vi "StateArm.vi"(0 "Master State In":T1(ring)) -> ()   [LabVIEW 2020]
doc: "This VI makes all of the decisions related to the Arm subsystem."
uses:
  <vilib>/Rock Robotics/WPI/DriverStation/WPI_DriverStationRobotMode2.ctl
  91f446a8-b483-4e57-bb67-dcd3392c5748.vi
  cc244f82-53a2-44a0-9b94-e9a7b6ef83dd.vi
  GlobalDriverStationCommands.vi
  GlobalPoseAndTargeting.vi
  GlobalDriverStationData.vi
  GlobalArm.vi
panel:
  out "Pre-Ground":cluster{dbl, dbl, dbl}
  in  "Pre-Ground Auto":cluster{dbl, dbl, dbl}={113.0, 144.0, 280.0}
  in  "Pre-Scoring Mid Cube":cluster{dbl, dbl, dbl}={90.0, 180.0, 180.0}
  in  "Pre-Scoring High Cube":cluster{dbl, dbl, dbl}={100.0, 270.0, 109.0}
  in  "Pre-Scoring Mid Cone":cluster{dbl, dbl, dbl}={90.0, 280.0, 90.0}
  in  "Pre-Scoring High Cone":cluster{dbl, dbl, dbl}={100.0, 275.0, 85.0}
  in  "Ground":cluster{dbl, dbl, dbl}={113.0, 144.0, 350.0}
  in  "Pre-Substation":cluster{dbl, dbl, dbl}={80.0, 149.0, 215.0}
  in  "Low Score Back":cluster{dbl, dbl, dbl}={90.0, 180.0, 155.0}
  in  "Low Score Front":cluster{dbl, dbl, dbl}={90.0, 180.0, 265.0}
  in  "Shelf":cluster{dbl, dbl, dbl}={104.0, 290.0, -72.0}
  in  "High Cube (IK)":cluster{dbl, dbl, dbl}={202.0, -50.7, 59.0}
  in  "Mid Cube (IK)":cluster{dbl, dbl, dbl}={210.0, -35.5, 50.0}
  in  "High Cone (IK)":cluster{dbl, dbl, dbl}={190.0, -53.0, 62.5}
  in  "Mid Cone (IK)":cluster{dbl, dbl, dbl}={180.0, -42.5, 51.7}
  in  "Pre-Shelf":cluster{dbl, dbl, dbl}={104.0, 309.0, -85.0}
  in  "Initial Scoring Guess":cluster{dbl, dbl, dbl}={100.0, 230.0, 125.0}
  out "Current Sequence Step":i32
  in  "Substation":cluster{dbl, dbl, dbl}={80.0, 149.0, 280.0}
  in  "Stowed":cluster{dbl, dbl, dbl}={90.0, 180.0, 180.0}
  in  "Pre-Ground Teleop":cluster{dbl, dbl, dbl}={113.0, 144.0, 180.0}
  out "You Have Arrived":bool
  out "Pre-Scoring":cluster{dbl, dbl, dbl}
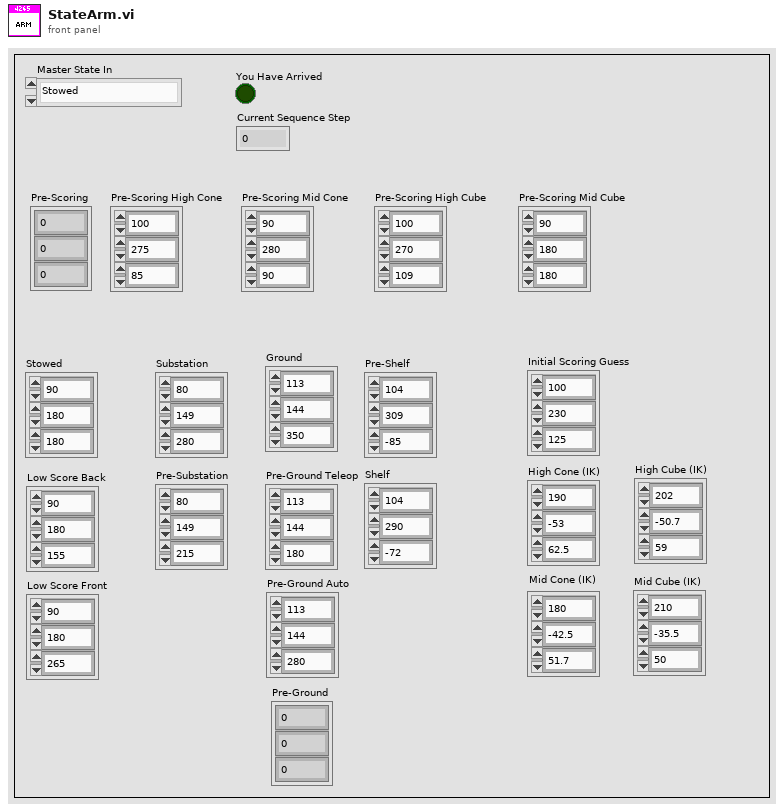
[diagram p1: front panel]
types:
  T1 = enum16{"Stowed", "Balancing", "Scoring", "Hoppering", "Ground", "Shelf"}
  T2 = typedef "WPI_DriverStationRobotMode2.ctl" = enum16{"Autonomous Disabled", "Autonomous Enabled", "Teleop Disabled", "Teleop Enabled", "Disconnected", "Finish", "Test Disabled", "Test Enabled", "Emergency Stopped"}
  T3 = enum16{"Low Cube", "Mid Cube", "High Cube", "Low Cone", "Mid Cone", "High Cone"}
  T4 = enum16{"Safety", "Travelling", "Positioning", "Holding"}
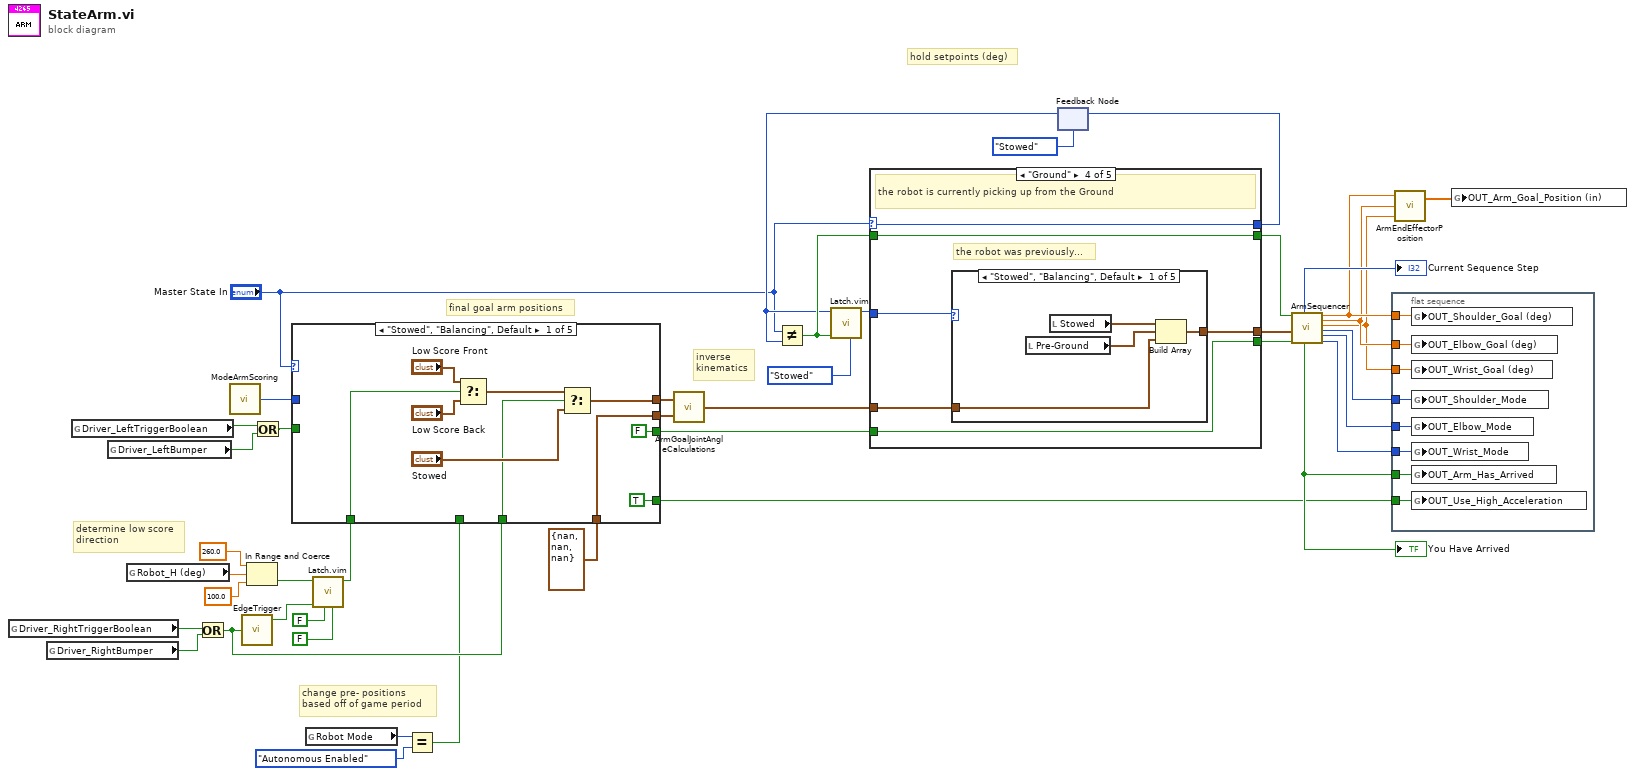
[diagram p0: block diagram]
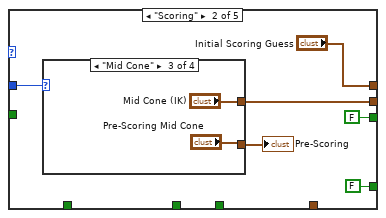
[diagram p2: hidden frame]
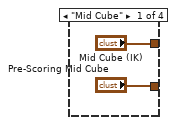
[diagram p3: hidden frame]
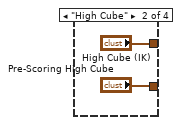
[diagram p4: hidden frame]
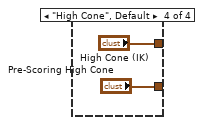
[diagram p5: hidden frame]
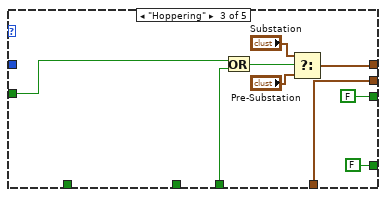
[diagram p6: hidden frame]
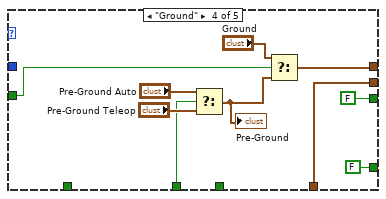
[diagram p7: hidden frame]
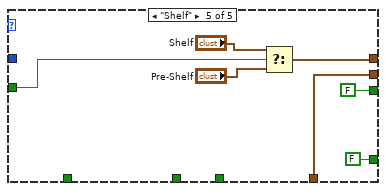
[diagram p8: hidden frame]
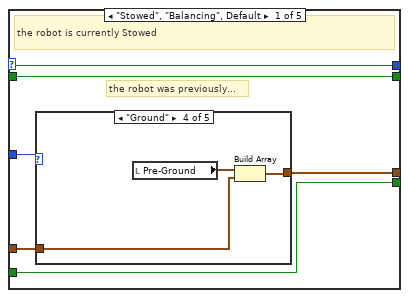
[diagram p9: hidden frame]
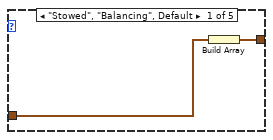
[diagram p10: hidden frame]
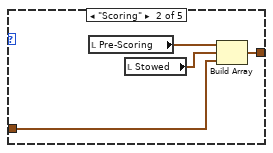
[diagram p11: hidden frame]
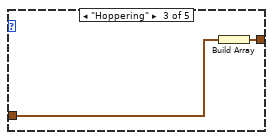
[diagram p12: hidden frame]
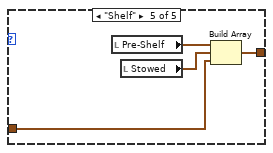
[diagram p13: hidden frame]
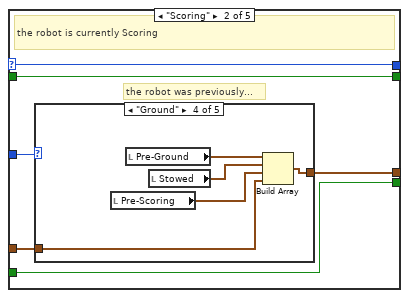
[diagram p14: hidden frame]
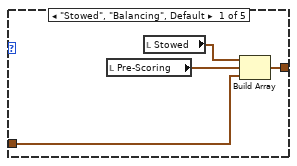
[diagram p15: hidden frame]
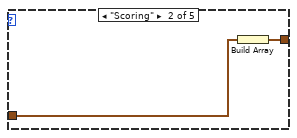
[diagram p16: hidden frame]
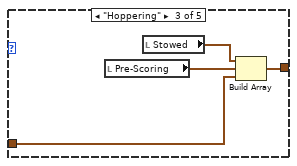
[diagram p17: hidden frame]
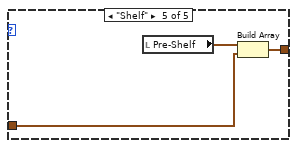
[diagram p18: hidden frame]
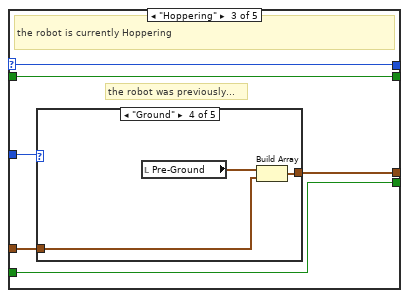
[diagram p19: hidden frame]
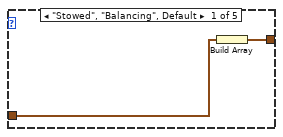
[diagram p20: hidden frame]
diagram:
  # "change pre- positions\nbased off of game period"
  # "determine low score\ndirection"
  # "inverse\nkinematics"
  # "hold setpoints (deg)"
  # "final goal arm positions"
  n1 = global read "GlobalDriverStationCommands.vi" "Driver_RightTriggerBoolean"() -> (w6:bool)
  n2 = global read "GlobalDriverStationCommands.vi" "Driver_RightBumper"() -> (w7:bool)
  n3 = global read "GlobalDriverStationCommands.vi" "Driver_LeftTriggerBoolean"() -> (w10:bool)
  n4 = global read "GlobalDriverStationCommands.vi" "Driver_LeftBumper"() -> (w9:bool)
  n5 = global read "GlobalPoseAndTargeting.vi" "Robot_H (deg)"() -> (w18:dbl)
  n6 = Or(x=w6, y=w7) -> (x .or. y?=w5:bool)
  n7 = call "ModeArmScoring.vi"() -> ("Scoring Position"=w28:T3)  [unwired: 1 in]
  n8 = call "EdgeTrigger.vi"("Input Signal"=w5) -> ("Rising Edge Trigger"=w12:bool)  [unwired: 2 out]
  n9 = In Range and Coerce(upper limit=260.0, x=w18, lower limit=100.0) -> (In Range?=w15:bool)  [unwired: 1 out]
  n10 = Or(x=w10, y=w9) -> (x .or. y?=w8:bool)
  n11 = global read "GlobalDriverStationData.vi" "Robot Mode"() -> (w4:T2)
  n12 = call "Latch.vim"("Default Value"=FALSE, "Reset"=FALSE, "Latch Signal"=w12, "Latch Value"=w15) -> ("Latched"=w11:bool)  [unwired: 7 in]
  n13 = Equal?(x=w4, y=WPI_DriverStationRobotMode2."Autonomous Enabled") -> (x = y?=w2:bool)
  n14 = case shown="\"Stowed\", \"Balancing\", Default" "Master State In" {
    tunnel: w28 -> [_ w59 _ _ _]
    tunnel: [w47 "Initial Scoring Guess" w73 w84 w89] -> w30
    tunnel: [w53 w58 w76 w86 w90] -> w27
    tunnel: cluster{dbl, dbl, dbl} {nan, nan, nan} ("PreShelf (IK)") -> [w53 _ w76 w86 w90]
    tunnel: [FALSE ("OUT_Hopper_Arm_Position") FALSE ("OUT_Hopper_Arm_Position") FALSE ("OUT_Hopper_Arm_Position") FALSE ("OUT_Hopper_Arm_Position") FALSE ("OUT_Hopper_Arm_Position")] -> w20
    tunnel: w11 -> [w46 _ _ _ _]
    tunnel: w5 -> [w45 _ w70 _ _]
    tunnel: w8 -> [_ _ w69 w82 w88]
    tunnel: w2 -> [_ _ _ w78 _]
    tunnel: [TRUE FALSE FALSE FALSE FALSE] -> w1
    frame "Stowed", "Balancing", Default {
      n15 = Select(t="Low Score Front", s=w46, f="Low Score Back") -> (s? t:f=w50:cluster{dbl, dbl, dbl})
      n16 = Select(t=w50, s=w45, f="Stowed") -> (s? t:f=w47:cluster{dbl, dbl, dbl})
    }
    frame "Scoring" {
      n17 = case shown="\"Mid Cone\"" w59 {
        tunnel: ["Mid Cube (IK)" "High Cube (IK)" "Mid Cone (IK)" "High Cone (IK)"] -> w58
        tunnel: ["Pre-Scoring Mid Cube" "Pre-Scoring High Cube" "Pre-Scoring Mid Cone" "Pre-Scoring High Cone"] -> w55
        frame "Mid Cube" {
        }
        frame "High Cube" {
        }
        frame "Mid Cone" {
        }
        frame "High Cone", Default {
        }
      }
      "Pre-Scoring" <- w55
    }
    frame "Hoppering" {
      n18 = Or(x=w69, y=w70) -> (x .or. y?=w71:bool)
      n19 = Select(t="Substation", s=w71, f="Pre-Substation") -> (s? t:f=w73:cluster{dbl, dbl, dbl})
    }
    frame "Ground" {
      n20 = Select(t="Pre-Ground Auto", s=w78, f="Pre-Ground Teleop") -> (s? t:f=w79:cluster{dbl, dbl, dbl})
      "Pre-Ground" <- w79
      n21 = Select(t="Ground", s=w82, f=w79) -> (s? t:f=w84:cluster{dbl, dbl, dbl})
    }
    frame "Shelf" {
      n22 = Select(t="Shelf", s=w88, f="Pre-Shelf") -> (s? t:f=w89:cluster{dbl, dbl, dbl})
    }
  }
  n23 = call "ArmGoalJointAngleCalculations.vi"("Goal End Effector Position"=w27, "Intial Joint Angle Guesses (deg)"=w30) -> ("Goal Joint Angles (deg)"=w29:cluster{dbl, dbl, dbl})  [unwired: 1 in]
  n24 = feedback #1(T1."Stowed" ("Master State In")) -> (w35:T1)
  n25 = Not Equal?(x="Master State In", y=w35) -> (x != y?=w36:bool)
  n26 = call "Latch.vim"("Default Value"=T1."Stowed" ("Master State In"), "Latch Signal"=w36, "Latch Value"=w35) -> ("Latched"=w41:T1)  [unwired: 8 in]
  n27 = case shown="\"Ground\"" "Master State In" {
    selector: "Master State In" -> [w99 w120 w144 w165 w190]
    tunnel: [w99 w120 w144 w165 w190] -> w43
    tunnel: w41 -> [w98 w119 w143 w164 w189]
    tunnel: w36 -> [w97 w116 w141 w163 w188]
    tunnel: w29 -> [w95 w118 w140 w161 w186]
    tunnel: [w96 w117 w142 w162 w187] -> w39
    tunnel: [w97 w116 w141 w163 w188] -> w37
    tunnel: [w94 w115 w139 w160 w185] -> w21
    tunnel: w20 -> [w94 w115 w139 w160 w185]
    frame "Stowed", "Balancing", Default {
      # "the robot was previously..."
      # "the robot is currently Stowed"
      n28 = case shown="\"Ground\"" w98 {
        tunnel: [w101 w105 w107 w110 w114] -> w96
        tunnel: w95 -> [w100 w104 w106 w109 w111]
        frame "Stowed", "Balancing", Default {
          n29 = Build Array(w100) -> (w101:cluster{dbl, dbl, dbl}[])
        }
        frame "Scoring" {
          n30 = local read "Pre-Scoring"() -> (w103:cluster{dbl, dbl, dbl})
          n31 = local read "Stowed"() -> (w102:cluster{dbl, dbl, dbl})
          n32 = Build Array(w103, w102, w104) -> (w105:cluster{dbl, dbl, dbl}[])
        }
        frame "Hoppering" {
          n33 = Build Array(w106) -> (w107:cluster{dbl, dbl, dbl}[])
        }
        frame "Ground" {
          n34 = local read "Pre-Ground"() -> (w108:cluster{dbl, dbl, dbl})
          n35 = Build Array(w108, w109) -> (w110:cluster{dbl, dbl, dbl}[])
        }
        frame "Shelf" {
          n36 = local read "Pre-Shelf"() -> (w113:cluster{dbl, dbl, dbl})
          n37 = local read "Stowed"() -> (w112:cluster{dbl, dbl, dbl})
          n38 = Build Array(w113, w112, w111) -> (w114:cluster{dbl, dbl, dbl}[])
        }
      }
    }
    frame "Scoring" {
      # "the robot was previously..."
      # "the robot is currently Scoring"
      n39 = case shown="\"Ground\"" w119 {
        tunnel: [w124 w126 w130 w134 w137] -> w117
        tunnel: w118 -> [w123 w125 w129 w135 w138]
        frame "Stowed", "Balancing", Default {
          n40 = local read "Pre-Scoring"() -> (w121:cluster{dbl, dbl, dbl})
          n41 = local read "Stowed"() -> (w122:cluster{dbl, dbl, dbl})
          n42 = Build Array(w122, w121, w123) -> (w124:cluster{dbl, dbl, dbl}[])
        }
        frame "Scoring" {
          n43 = Build Array(w125) -> (w126:cluster{dbl, dbl, dbl}[])
        }
        frame "Hoppering" {
          n44 = local read "Pre-Scoring"() -> (w128:cluster{dbl, dbl, dbl})
          n45 = local read "Stowed"() -> (w127:cluster{dbl, dbl, dbl})
          n46 = Build Array(w127, w128, w129) -> (w130:cluster{dbl, dbl, dbl}[])
        }
        frame "Ground" {
          n47 = local read "Pre-Scoring"() -> (w133:cluster{dbl, dbl, dbl})
          n48 = local read "Pre-Ground"() -> (w132:cluster{dbl, dbl, dbl})
          n49 = local read "Stowed"() -> (w131:cluster{dbl, dbl, dbl})
          n50 = Build Array(w132, w131, w133, w135) -> (w134:cluster{dbl, dbl, dbl}[])
        }
        frame "Shelf" {
          n51 = local read "Pre-Shelf"() -> (w136:cluster{dbl, dbl, dbl})
          n52 = Build Array(w136, w138) -> (w137:cluster{dbl, dbl, dbl}[])
        }
      }
    }
    frame "Hoppering" {
      # "the robot was previously..."
      # "the robot is currently Hoppering"
      n53 = case shown="\"Ground\"" w143 {
        tunnel: [w146 w150 w152 w155 w159] -> w142
        tunnel: w140 -> [w145 w149 w151 w154 w158]
        frame "Stowed", "Balancing", Default {
          n54 = Build Array(w145) -> (w146:cluster{dbl, dbl, dbl}[])
        }
        frame "Scoring" {
          n55 = local read "Pre-Scoring"() -> (w148:cluster{dbl, dbl, dbl})
          n56 = local read "Stowed"() -> (w147:cluster{dbl, dbl, dbl})
          n57 = Build Array(w148, w147, w149) -> (w150:cluster{dbl, dbl, dbl}[])
        }
        frame "Hoppering" {
          n58 = Build Array(w151) -> (w152:cluster{dbl, dbl, dbl}[])
        }
        frame "Ground" {
          n59 = local read "Pre-Ground"() -> (w153:cluster{dbl, dbl, dbl})
          n60 = Build Array(w153, w154) -> (w155:cluster{dbl, dbl, dbl}[])
        }
        frame "Shelf" {
          n61 = local read "Pre-Shelf"() -> (w157:cluster{dbl, dbl, dbl})
          n62 = local read "Stowed"() -> (w156:cluster{dbl, dbl, dbl})
          n63 = Build Array(w157, w156, w158) -> (w159:cluster{dbl, dbl, dbl}[])
        }
      }
    }
    frame "Ground" {
      # "the robot was previously..."
      # "the robot is currently picking up from the Ground"
      n64 = case shown="\"Stowed\", \"Balancing\", Default" w164 {
        tunnel: [w169 w174 w177 w178 w184] -> w162
        tunnel: w161 -> [w168 w170 w176 w179 w182]
        frame "Stowed", "Balancing", Default {
          n65 = local read "Pre-Ground"() -> (w166:cluster{dbl, dbl, dbl})
          n66 = local read "Stowed"() -> (w167:cluster{dbl, dbl, dbl})
          n67 = Build Array(w167, w166, w168) -> (w169:cluster{dbl, dbl, dbl}[])
        }
        frame "Scoring" {
          n68 = local read "Pre-Scoring"() -> (w173:cluster{dbl, dbl, dbl})
          n69 = local read "Pre-Ground"() -> (w171:cluster{dbl, dbl, dbl})
          n70 = local read "Stowed"() -> (w172:cluster{dbl, dbl, dbl})
          n71 = Build Array(w173, w172, w171, w170) -> (w174:cluster{dbl, dbl, dbl}[])
        }
        frame "Hoppering" {
          n72 = local read "Pre-Ground"() -> (w175:cluster{dbl, dbl, dbl})
          n73 = Build Array(w175, w176) -> (w177:cluster{dbl, dbl, dbl}[])
        }
        frame "Ground" {
          n74 = Build Array(w179) -> (w178:cluster{dbl, dbl, dbl}[])
        }
        frame "Shelf" {
          n75 = local read "Pre-Ground"() -> (w183:cluster{dbl, dbl, dbl})
          n76 = local read "Pre-Shelf"() -> (w181:cluster{dbl, dbl, dbl})
          n77 = local read "Stowed"() -> (w180:cluster{dbl, dbl, dbl})
          n78 = Build Array(w181, w180, w183, w182) -> (w184:cluster{dbl, dbl, dbl}[])
        }
      }
    }
    frame "Shelf" {
      # "the robot was previously...."
      # "the robot is currently picking up from the Shelf"
      n79 = case shown="\"Ground\"" w189 {
        tunnel: [w194 w197 w201 w206 w208] -> w187
        tunnel: w186 -> [w193 w196 w200 w205 w207]
        frame "Stowed", "Balancing", Default {
          n80 = local read "Pre-Shelf"() -> (w191:cluster{dbl, dbl, dbl})
          n81 = local read "Stowed"() -> (w192:cluster{dbl, dbl, dbl})
          n82 = Build Array(w192, w191, w193) -> (w194:cluster{dbl, dbl, dbl}[])
        }
        frame "Scoring" {
          n83 = local read "Pre-Shelf"() -> (w195:cluster{dbl, dbl, dbl})
          n84 = Build Array(w195, w196) -> (w197:cluster{dbl, dbl, dbl}[])
        }
        frame "Hoppering" {
          n85 = local read "Stowed"() -> (w198:cluster{dbl, dbl, dbl})
          n86 = local read "Pre-Shelf"() -> (w199:cluster{dbl, dbl, dbl})
          n87 = Build Array(w198, w199, w200) -> (w201:cluster{dbl, dbl, dbl}[])
        }
        frame "Ground" {
          n88 = local read "Pre-Ground"() -> (w203:cluster{dbl, dbl, dbl})
          n89 = local read "Pre-Shelf"() -> (w204:cluster{dbl, dbl, dbl})
          n90 = local read "Stowed"() -> (w202:cluster{dbl, dbl, dbl})
          n91 = Build Array(w203, w202, w204, w205) -> (w206:cluster{dbl, dbl, dbl}[])
        }
        frame "Shelf" {
          n92 = Build Array(w207) -> (w208:cluster{dbl, dbl, dbl}[])
        }
      }
    }
  }
  n93 = feedback-in #1(w43) -> ()
  n94 = call "ArmSequencer.vi"("Reset"=w37, "Array of Arm Joint Goals"=w39, "Treat Wrist as Four-Bar"=w21) -> ("Current Sequence Step"=→"Current Sequence Step":i32, "Arm Has Arrived"=w19:bool, "Goal Shoulder Angle (deg)"=w33:dbl, "Goal Elbow Angle (deg)"=w32:dbl, "Goal Wrist Angle (deg)"=w31:dbl, "Shoulder Control Mode"=w24:T4, "Elbow Control Mode"=w23:T4, "Wrist Control Mode"=w22:T4)  [unwired: 9 in]
  "You Have Arrived" <- w19
  n95 = flat-sequence {
    tunnel: w33 -> [w216]
    tunnel: w32 -> [w215]
    tunnel: w31 -> [w214]
    tunnel: w24 -> [w213]
    tunnel: w23 -> [w212]
    tunnel: w22 -> [w211]
    tunnel: w19 -> [w210]
    tunnel: w1 -> [w209]
    frame #0 {
      n96 = global write "GlobalArm.vi" "OUT_Shoulder_Goal (deg)"(w216) -> ()
      n97 = global write "GlobalArm.vi" "OUT_Elbow_Goal (deg)"(w215) -> ()
      n98 = global write "GlobalArm.vi" "OUT_Wrist_Goal (deg)"(w214) -> ()
      n99 = global write "GlobalArm.vi" "OUT_Shoulder_Mode"(w213) -> ()
      n100 = global write "GlobalArm.vi" "OUT_Elbow_Mode"(w212) -> ()
      n101 = global write "GlobalArm.vi" "OUT_Wrist_Mode"(w211) -> ()
      n102 = global write "GlobalArm.vi" "OUT_Arm_Has_Arrived"(w210) -> ()
      n103 = global write "GlobalArm.vi" "OUT_Use_High_Acceleration"(w209) -> ()
    }
  }
  n104 = call "ArmEndEffectorPosition.vi"("Wrist Angle (deg)"=w31, "Elbow Angle (deg)"=w32, "Shoulder Angle (deg)"=w33) -> ("Translation Vector (in)"=w34:dbl[])  [unwired: 1 out]
  n105 = global write "GlobalArm.vi" "OUT_Arm_Goal_Position (in)"(w34) -> ()
